vi "Periodic Tasks.vi"(8 "error in":errorcluster) -> ()   [LabVIEW 2014]
doc: "This VI runs in parallel to other tasks. It can contain as many user-defined periodic loops as you need. These can carry out PID or other sorts of timed response."
uses:
  <vilib>/Rock Robotics/SystemInterfaces/Utilities/FPGA_UtilitiesLED Source.ctl
  <vilib>/Rock Robotics/SystemInterfaces/Utilities/FPGA_UtilitiesLED State.ctl
  Robot Global Data.vi
  <vilib>/Rock Robotics/WPI/Relay/WPI_RelayValue.ctl
panel:
  out "Encoder Alarm Statuses":string[](array[string])
  out "Directions":string[](array[string])
  out "Velocities":dbl[](array[numeric])
  out "Encoder Distances":dbl[](array[numeric])
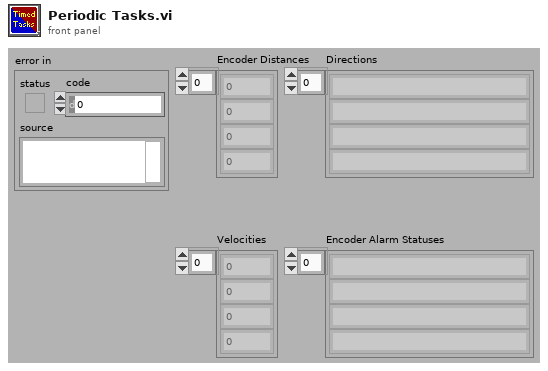
[diagram p1: front panel]
types:
  T1 = enum16{"open", "replace", "create", "open or create", "replace or create", "replace or create with confirmation"}
  T2 = typedef "WPI_DigitalInputDevRef.ctl" = cluster{"DevStatus":errorcluster, "DIO Channel":T3, "Digital Module":T4}
  T3 = typedef "FPGA_DIOChannel.ctl" = enum8{"DIO 1", "DIO 2", "DIO 3", "DIO 4", "DIO 5", "DIO 6", "DIO 7", "DIO 8", "DIO 9", "DIO 10", "DIO 11", "DIO 12", "DIO 13", "DIO 14", "Invalid"}
  T4 = typedef "FPGA_TypedefDigitalModule.ctl" = enum16{"Digital Module 1", "Digital Module 2"}
  T5 = typedef "WPI_RelayValue.ctl" = enum16{"Off", "On", "Forward", "Reverse"}
  T6 = typedef "WPI_RelayDevRef.ctl" = cluster{"DevStatus":errorcluster, "Relay Channel":T7, "Digital Module":T4, "Relay Direction":T8}
  T7 = typedef "FPGA_DIORelayChannel.ctl" = enum8{"Relay 1", "Relay 2", "Relay 3", "Relay 4", "Relay 5", "Relay 6", "Relay 7", "Relay 8", "Invalid"}
  T8 = typedef "WPI_RelayDirection.ctl" = enum16{"Both directions", "Forward only", "Reverse only"}
  T9 = typedef "FPGA_UtilitiesLED State.ctl" = enum16{"Off", "On", "Toggle"}
  T10 = typedef "FPGA_UtilitiesLED Source.ctl" = enum16{"User LED", "FPGA LED"}
  T11 = typedef "WPI_AnalogChannelDevRef.ctl" = cluster{"DevStatus":errorcluster, "Analog Module":T12, "Analog Channel":T13}
  T12 = typedef "FPGA_TypedefAnalogModule.ctl" = enum16{"Analog Module 1", "Analog Module 2"}
  T13 = typedef "FPGA_AIChannel.ctl" = enum8{"AI 1", "AI 2", "AI 3", "AI 4", "AI 5", "AI 6", "AI 7", "AI 8", "Invalid"}
  T14 = typedef "WPI_GyroDevRef.ctl" = cluster{"DevStatus":errorcluster, "Analog Module":T12, "Analog Channel":T13, "Offset":dbl, "Gain (VoltsPerDegree/Second)":dbl}
  T15 = typedef "WPI_CompressorDevRef.ctl" = cluster{"DevStatus":errorcluster, "DigitalInputDevRef":T2, "RelayDevRef":T6}
  T16 = typedef "WPI_EncoderDevRef.ctl" = cluster{"DevStatus":errorcluster, "EncoderIndex":T17, "CounterIndex":T18, "DistancePerCount":dbl, "Decoding Type":T19}
  T17 = typedef "FPGA_EncoderIdx.ctl" = enum8{"Enc 0", "Enc 1", "Enc 2", "Enc 3", "Invalid"}
  T18 = typedef "FPGA_CounterCtrSystemIndex.ctl" = enum8{"Ctr 0", "Ctr 1", "Ctr 2", "Ctr 3", "Ctr 4", "Ctr 5", "Ctr 6", "Ctr 7", "Invalid"}
  T19 = typedef "WPI_EncoderType.ctl" = enum16{"1x", "2x", "4x"}
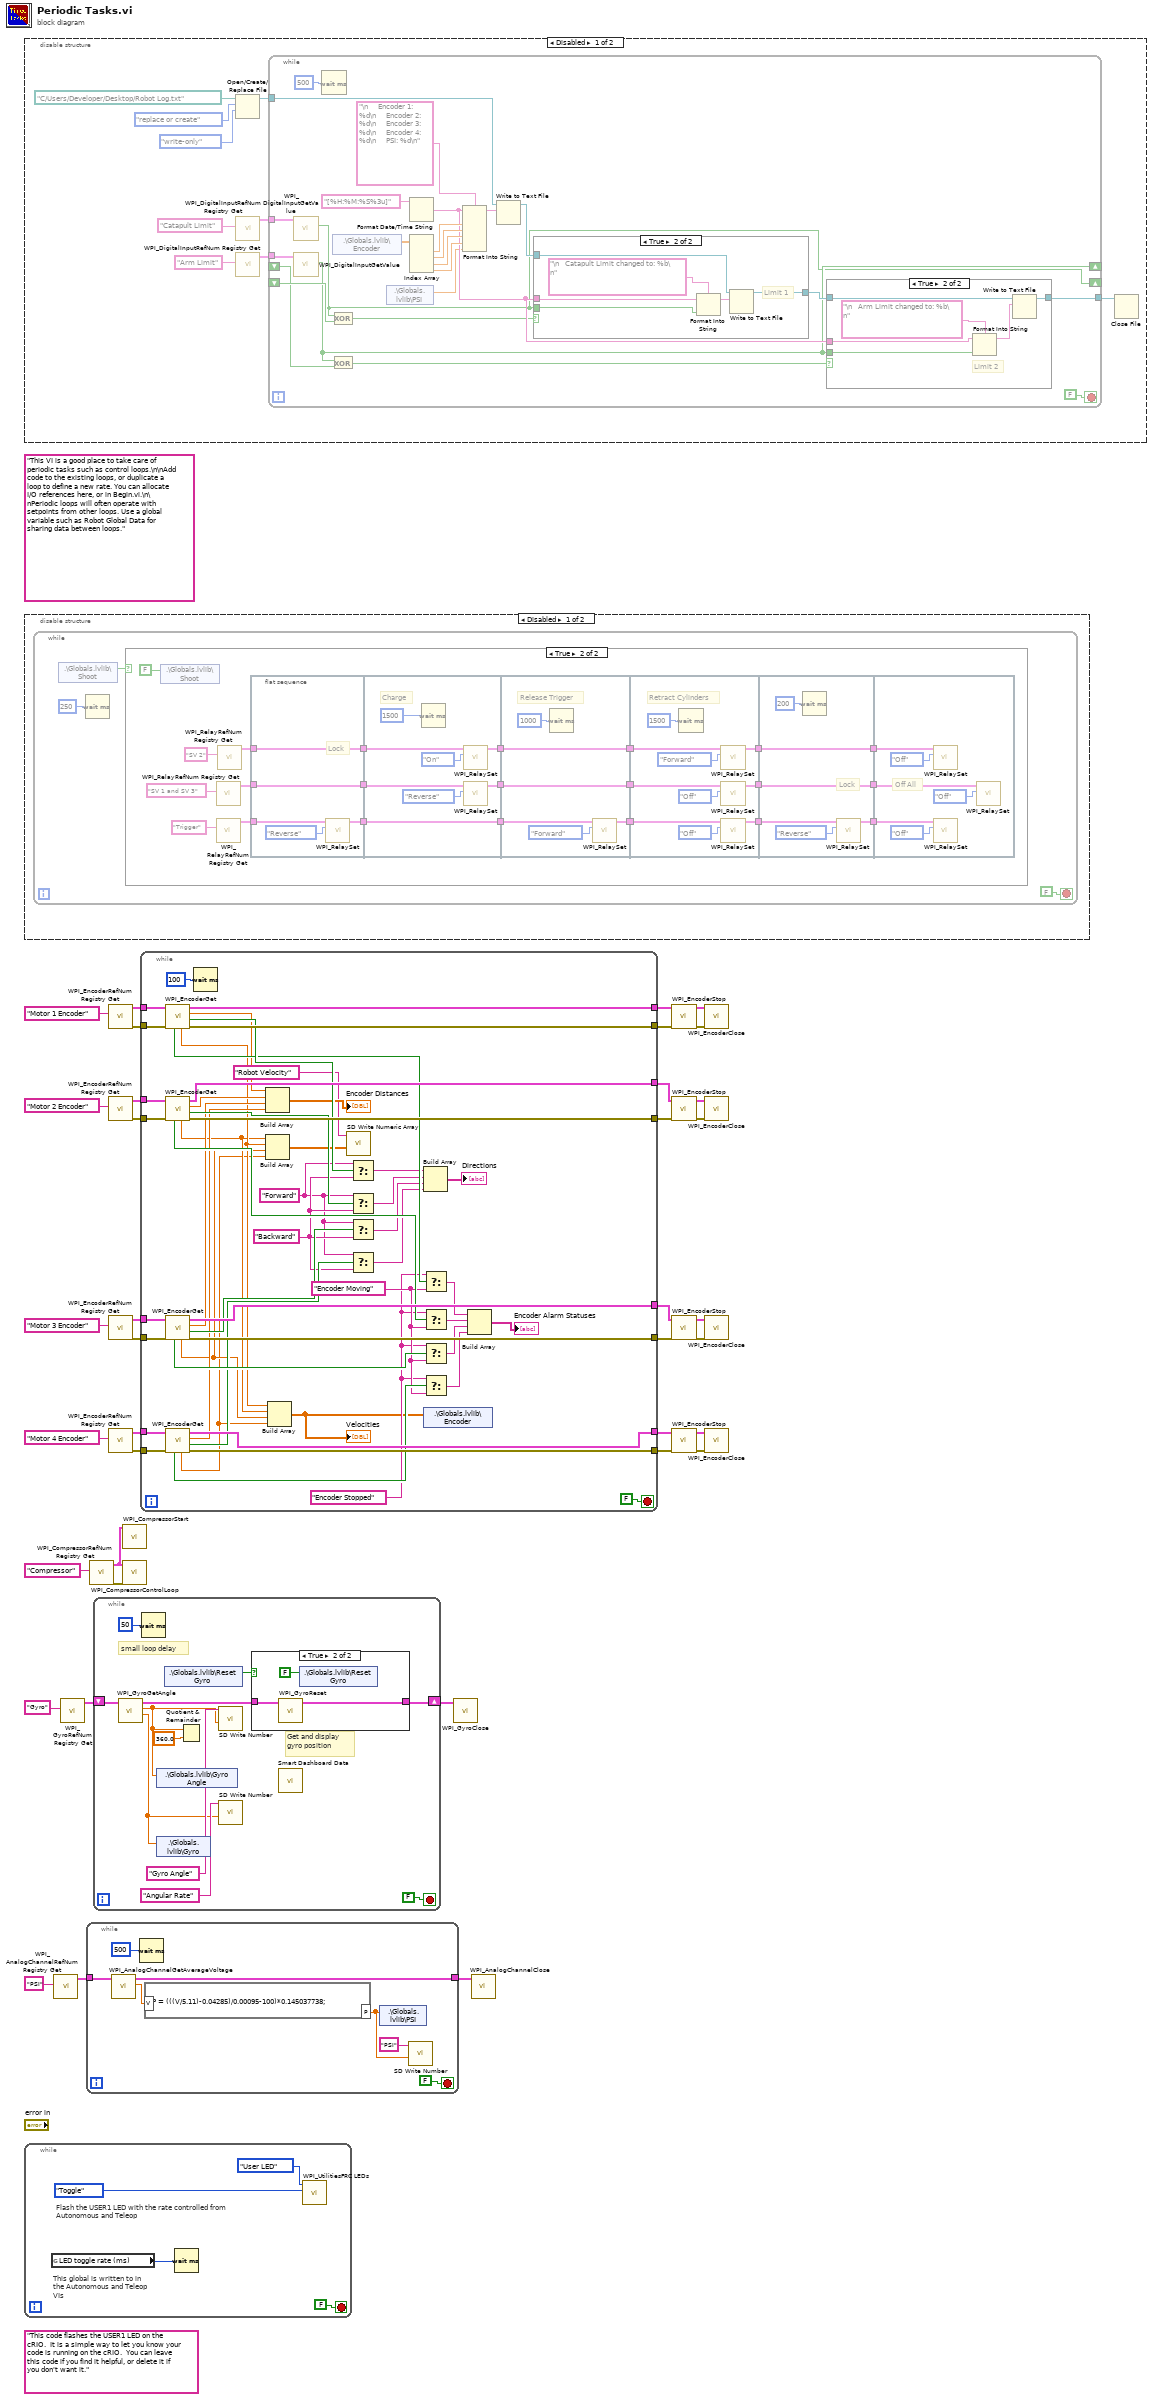
[diagram p0: block diagram]
diagram:
  (unwired) "This code flashes the USER1 LED on the cRIO.  It is a simple way to let you know your code is running on the cRIO.  You can leave this code if you find it helpful, or delete it if you don't want it."
  (unwired) "This VI is a good place to take care of periodic tasks such as control loops.\n\nAdd code to the existing loops, or duplicate a loop to define a new rate. You can allocate I/O references here, or in Begin.vi.\n\nPeriodic loops will often operate with setpoints from other loops. Use a global variable such as Robot Global Data for sharing data between loops."
  n1 = disable-structure shown="Disabled" {
    frame Disabled {
      n2 = Open/Create/Replace File(file path (use dialog)=path "C:/Users/Developer/Desktop/Robot Log.txt", operation (0:open)=T1."replace or create", access (0:read/write)=enum16{"read/write", "read-only", "write-only"}."write-only") -> (refnum out=w43:refnum<file>)  [unwired: 3 in, 2 out]
      n3 = call <vilib>:"WPI_DigitalInputRefNum Registry Get.vi"("refnum name"="Catapult Limit") -> ("DigitalInputDevRef"=w38:T2)  [unwired: 9 in, 1 out]
      n4 = call <vilib>:"WPI_DigitalInputRefNum Registry Get.vi"("refnum name"="Arm Limit") -> ("DigitalInputDevRef"=w39:T2)  [unwired: 9 in, 1 out]
      n5 = while {
        tunnel: w43 -> [w66]
        tunnel: [w55] -> w42
        shift-right: [w51] -> _
        shift-left: _ -> [w58]
        shift-right: [w50] -> _
        shift-left: _ -> [w59]
        tunnel: w39 -> [w49]
        tunnel: w38 -> [w48]
        stop <- FALSE stop-if-true
        n6 = call <vilib>:"WPI_DigitalInputGetValue.vi"("DigitalInputDevRef"=w48) -> ("Value"=w50:bool)  [unwired: 8 in, 2 out]
        n7 = call <vilib>:"WPI_DigitalInputGetValue.vi"("DigitalInputDevRef"=w49) -> ("Value"=w51:bool)  [unwired: 8 in, 2 out]
        n8 = Wait (ms)(milliseconds to wait=u32 500) -> ()  [unwired: 1 out]
        n9 = Exclusive Or(1:w59, 2:w50) -> (0:w53:bool)
        n10 = Exclusive Or(1:w58, 2:w51) -> (0:w52:bool)
        n11 = shared-variable ".\\Globals.lvlib\\Encoder"() -> (w64:dbl[])  [unwired: 1 in, 1 out]
        n12 = shared-variable ".\\Globals.lvlib\\PSI"() -> (w47:dbl)  [unwired: 1 in, 1 out]
        n13 = Format Date/Time String(time format string (%c)="[%H:%M:%S%3u]") -> (date/time string=w54:string)  [unwired: 2 in]
        n14 = Index Array(array=w64) -> (element #1=w63:dbl, element #2=w62:dbl, element #3=w61:dbl, element #4=w60:dbl)  [unwired: 4 in]
        n15 = Format Into String(format string="\n     Encoder 1: %d\n     Encoder 2: %d\n     Encoder 3: %d\n     Encoder 4: %d\n     PSI: %d\n", initial string=w54, w63, w62, w61, w60, w47) -> (resulting string=w67:string)  [unwired: 1 in, 1 out]
        n16 = Write to Text File(file (use dialog)=w66, text=w67) -> (refnum out=w57:refnum<file>)  [unwired: 2 in, 2 out]
        n17 = case shown="True" w53 {
          tunnel: w50 -> [_ w84]
          tunnel: w57 -> [w78 w83]
          tunnel: [w78 w82] -> w56
          tunnel: w54 -> [_ w81]
          frame False {
          }
          frame True {
            # "Limit 1"
            n18 = Format Into String(format string="\n   Catapult Limit changed to: %b\n", initial string=w81, w84) -> (resulting string=w79:string)  [unwired: 1 in, 1 out]
            n19 = Write to Text File(file (use dialog)=w83, text=w79) -> (refnum out=w82:refnum<file>)  [unwired: 2 in, 2 out]
          }
        }
        n20 = case shown="True" w52 {
          tunnel: w51 -> [_ w77]
          tunnel: w56 -> [w71 w76]
          tunnel: [w71 w75] -> w55
          tunnel: w54 -> [_ w74]
          frame False {
          }
          frame True {
            # "Limit 2"
            n21 = Format Into String(format string="\n   Arm Limit changed to: %b\n", initial string=w74, w77) -> (resulting string=w72:string)  [unwired: 1 in, 1 out]
            n22 = Write to Text File(file (use dialog)=w76, text=w72) -> (refnum out=w75:refnum<file>)  [unwired: 2 in, 2 out]
          }
        }
      }
      n23 = Close File(refnum=w42) -> ()  [unwired: 1 in, 2 out]
    }
    frame Enabled {
    }
  }
  n24 = disable-structure shown="Disabled" {
    frame Disabled {
      n25 = while {
        stop <- FALSE stop-if-true
        n26 = shared-variable ".\\Globals.lvlib\\Shoot"() -> (w86:bool)  [unwired: 1 in, 1 out]
        n27 = Wait (ms)(milliseconds to wait=u32 250) -> ()  [unwired: 1 out]
        n28 = case shown="True" w86 {
          frame False {
          }
          frame True {
            n29 = shared-variable ".\\Globals.lvlib\\Shoot"(FALSE ("Shoot")) -> ()  [unwired: 1 in, 1 out]
            n30 = call <vilib>:"WPI_RelayRefNum Registry Get.vi"("refnum name"="SV 1 and SV 3") -> ("RelayDevRef"=w104:T6)  [unwired: 9 in, 1 out]
            n31 = call <vilib>:"WPI_RelayRefNum Registry Get.vi"("refnum name"="Trigger") -> ("RelayDevRef"=w105:T6)  [unwired: 9 in, 1 out]
            n32 = call <vilib>:"WPI_RelayRefNum Registry Get.vi"("refnum name"="SV 2") -> ("RelayDevRef"=w106:T6)  [unwired: 9 in, 1 out]
            n33 = flat-sequence {
              tunnel: w106 -> [w112]
              tunnel: w105 -> [w113]
              tunnel: w104 -> [w111]
              tunnel: [w112] -> w103
              tunnel: [w111] -> w102
              tunnel: [w110] -> w101
              tunnel: w103 -> [w121]
              tunnel: w102 -> [w119]
              tunnel: w101 -> [w118]
              tunnel: [w118] -> w100
              tunnel: [w116] -> w98
              tunnel: [w115] -> w96
              tunnel: w100 -> [w127]
              tunnel: [w125] -> w99
              tunnel: w98 -> [w124]
              tunnel: [w124] -> w97
              tunnel: w96 -> [w123]
              tunnel: [w123] -> w95
              tunnel: w99 -> [w136]
              tunnel: w97 -> [w134]
              tunnel: w95 -> [w132]
              tunnel: [w131] -> w94
              tunnel: [w130] -> w93
              tunnel: [w129] -> w90
              tunnel: w94 -> [w144]
              tunnel: w93 -> [w142]
              tunnel: [w142] -> w92
              tunnel: [w141] -> w91
              tunnel: w90 -> [w141]
              tunnel: [w140] -> w89
              tunnel: w92 -> [w147]
              tunnel: w91 -> [w146]
              tunnel: w89 -> [w145]
              frame #0 {
                # "Lock"
                n34 = call <vilib>:"WPI_RelaySet.vi"("RelayValue"=WPI_RelayValue."Reverse", "RelayDevRef"=w113) -> ("RelayDevRef"=w110:T6)  [unwired: 8 in, 1 out]
              }
              frame #1 {
                # "Charge"
                n35 = Wait (ms)(milliseconds to wait=u32 1500) -> ()  [unwired: 1 out]
                n36 = call <vilib>:"WPI_RelaySet.vi"("RelayValue"=WPI_RelayValue."On", "RelayDevRef"=w121) -> ("RelayDevRef"=w115:T6)  [unwired: 8 in, 1 out]
                n37 = call <vilib>:"WPI_RelaySet.vi"("RelayValue"=WPI_RelayValue."Reverse", "RelayDevRef"=w119) -> ("RelayDevRef"=w116:T6)  [unwired: 8 in, 1 out]
              }
              frame #2 {
                # "Release Trigger"
                n38 = Wait (ms)(milliseconds to wait=u32 1000) -> ()  [unwired: 1 out]
                n39 = call <vilib>:"WPI_RelaySet.vi"("RelayValue"=WPI_RelayValue."Forward", "RelayDevRef"=w127) -> ("RelayDevRef"=w125:T6)  [unwired: 8 in, 1 out]
              }
              frame #3 {
                # "Retract Cylinders"
                n40 = Wait (ms)(milliseconds to wait=u32 1500) -> ()  [unwired: 1 out]
                n41 = call <vilib>:"WPI_RelaySet.vi"("RelayValue"=WPI_RelayValue."Forward", "RelayDevRef"=w132) -> ("RelayDevRef"=w129:T6)  [unwired: 8 in, 1 out]
                n42 = call <vilib>:"WPI_RelaySet.vi"("RelayValue"=WPI_RelayValue."Off", "RelayDevRef"=w134) -> ("RelayDevRef"=w130:T6)  [unwired: 8 in, 1 out]
                n43 = call <vilib>:"WPI_RelaySet.vi"("RelayValue"=WPI_RelayValue."Off", "RelayDevRef"=w136) -> ("RelayDevRef"=w131:T6)  [unwired: 8 in, 1 out]
              }
              frame #4 {
                # "Lock"
                n44 = Wait (ms)(milliseconds to wait=u32 200) -> ()  [unwired: 1 out]
                n45 = call <vilib>:"WPI_RelaySet.vi"("RelayValue"=WPI_RelayValue."Reverse", "RelayDevRef"=w144) -> ("RelayDevRef"=w140:T6)  [unwired: 8 in, 1 out]
              }
              frame #5 {
                # "Off All"
                n46 = call <vilib>:"WPI_RelaySet.vi"("RelayValue"=WPI_RelayValue."Off", "RelayDevRef"=w146) -> ()  [unwired: 8 in, 2 out]
                n47 = call <vilib>:"WPI_RelaySet.vi"("RelayValue"=WPI_RelayValue."Off", "RelayDevRef"=w145) -> ()  [unwired: 8 in, 2 out]
                n48 = call <vilib>:"WPI_RelaySet.vi"("RelayValue"=WPI_RelayValue."Off", "RelayDevRef"=w147) -> ()  [unwired: 8 in, 2 out]
              }
            }
          }
        }
      }
    }
    frame Enabled {
    }
  }
  n49 = while {
    stop <- FALSE stop-if-true
    # "This global is written to in the Autonomous and Teleop VIs"
    # "Flash the USER1 LED with the rate controlled from Autonomous and Teleop"
    n50 = global read "Robot Global Data.vi" "LED toggle rate (ms)"() -> (w151:u32)
    n51 = Wait (ms)(milliseconds to wait=w151) -> ()  [unwired: 1 out]
    n52 = call <vilib>:"WPI_UtilitiesFRC LEDs.vi"("State"=FPGA_UtilitiesLED_State."Toggle", "LED Type"=FPGA_UtilitiesLED_Source."User LED") -> ()  [unwired: 1 in, 9 out]
  }
  n53 = call <vilib>:"WPI_AnalogChannelRefNum Registry Get.vi"("refnum name"="PSI") -> ("AIDeviceRef"=w2:T11)  [unwired: 9 in, 1 out]
  n54 = call <vilib>:"WPI_GyroRefNum Registry Get.vi"("refnum name"="Gyro") -> ("GyroDevRef"=w37:T14)  [unwired: 9 in, 1 out]
  n55 = while {
    tunnel: w2 -> [w160]
    tunnel: [w156] -> w1
    stop <- FALSE stop-if-true
    n56 = call <vilib>:"WPI_AnalogChannelGetAverageVoltage.vi"("AIDeviceRef"=w160) -> ("Voltage"=w159:dbl, "AIDeviceRef"=w156:T11)  [unwired: 8 in, 1 out]
    n57 = Wait (ms)(milliseconds to wait=u32 500) -> ()  [unwired: 1 out]
    n58 = formula code="P = (((V/5.11)-0.04285)/0.00095-100)*0.145037738;"("V"=w159) -> ("P"=w157:dbl)
    n59 = shared-variable ".\\Globals.lvlib\\PSI"(w157) -> ()  [unwired: 1 in, 1 out]
    n60 = call <vilib>:"SD Write Number.vi"("Numeric"=w157, "Name"="PSI") -> ()  [unwired: 8 in, 2 out]
  }
  n61 = call <vilib>:"WPI_CompressorRefNum Registry Get.vi"("refnum name"="Compressor") -> ("error out"=w5:errorcluster, "CompressorDevRef"=w6:T15)  [unwired: 9 in]
  n62 = while {
    shift-right: [w167] -> w35
    shift-left: w37 -> [w169]
    stop <- FALSE stop-if-true
    # "small loop delay"
    # "Get and display\ngyro position"
    n63 = call <vilib>:"WPI_GyroGetAngle.vi"("GyroDevRef"=w169) -> ("Angular Rate"=w163:dbl, "Angle"=w162:dbl, "GyroDevRef"=w168:T14)  [unwired: 1 in, 7 out]
    n64 = Wait (ms)(milliseconds to wait=u32 50) -> ()  [unwired: 1 out]
    n65 = shared-variable ".\\Globals.lvlib\\Gyro Angle"(w162) -> ()  [unwired: 1 in, 1 out]
    n66 = shared-variable ".\\Globals.lvlib\\Gyro"(w163) -> ()  [unwired: 1 in, 1 out]
    n67 = shared-variable ".\\Globals.lvlib\\Reset Gyro"() -> (w166:bool)  [unwired: 1 in, 1 out]
    n68 = Quotient & Remainder(x=w162, y=360.0) -> ()  [unwired: 2 out]
    n69 = call <vilib>:"SD Write Number.vi"("Numeric"=w162, "Name"="Gyro Angle") -> ()  [unwired: 8 in, 2 out]
    n70 = call <vilib>:"SD Write Number.vi"("Numeric"=w163, "Name"="Angular Rate") -> ()  [unwired: 8 in, 2 out]
    n71 = case shown="True" w166 {
      tunnel: w168 -> [w173 w176]
      tunnel: [w173 w175] -> w167
      frame False {
      }
      frame True {
        n72 = call <vilib>:"WPI_GyroReset.vi"("GyroDevRef"=w176) -> ("GyroDevRef"=w175:T14)  [unwired: 9 in, 1 out]
        n73 = shared-variable ".\\Globals.lvlib\\Reset Gyro"(FALSE ("Reset Gyro")) -> ()  [unwired: 1 in, 1 out]
      }
    }
    n74 = call "Smart Dashboard Data.vi"() -> ()  [unwired: 12 in]
  }
  n75 = call <vilib>:"WPI_EncoderRefNum Registry Get.vi"("refnum name"="Motor 1 Encoder") -> ("error out"=w33:errorcluster, "EncoderDevRef"=w34:T16)  [unwired: 9 in]
  n76 = call <vilib>:"WPI_EncoderRefNum Registry Get.vi"("refnum name"="Motor 2 Encoder") -> ("error out"=w30:errorcluster, "EncoderDevRef"=w29:T16)  [unwired: 9 in]
  n77 = call <vilib>:"WPI_EncoderRefNum Registry Get.vi"("refnum name"="Motor 3 Encoder") -> ("error out"=w27:errorcluster, "EncoderDevRef"=w28:T16)  [unwired: 9 in]
  n78 = call <vilib>:"WPI_EncoderRefNum Registry Get.vi"("refnum name"="Motor 4 Encoder") -> ("error out"=w8:errorcluster, "EncoderDevRef"=w7:T16)  [unwired: 9 in]
  n79 = call <vilib>:"WPI_CompressorStart.vi"("CompressorDevRef"=w6) -> ()  [unwired: 9 in, 2 out]
  n80 = call <vilib>:"WPI_CompressorControlLoop.vi"("error in (no error)"=w5, "CompressorDevRef"=w6) -> ()  [unwired: 10 in]
  n81 = while {
    tunnel: w34 -> [w228]
    tunnel: w33 -> [w227]
    tunnel: w30 -> [w226]
    tunnel: w29 -> [w225]
    tunnel: w28 -> [w224]
    tunnel: w27 -> [w223]
    tunnel: [w222] -> w25
    tunnel: [w221] -> w22
    tunnel: [w220] -> w18
    tunnel: [w219] -> w17
    tunnel: [w218] -> w16
    tunnel: [w217] -> w14
    tunnel: [w216] -> w13
    tunnel: [w215] -> w10
    tunnel: w8 -> [w214]
    tunnel: w7 -> [w213]
    stop <- FALSE stop-if-true
    w201 = "Backward" ("f")
    w202 = "Encoder Moving" ("f")
    w199 = "Encoder Stopped"
    w200 = "Forward"
    n82 = call <vilib>:"WPI_EncoderGet.vi"("error in (no error)"=w227, "EncoderDevRef"=w228) -> ("error out"=w220:errorcluster, "Direction"=w207:bool, "Distance"=w198:dbl, "EncoderDevRef"=w222:T16, "Rate"=w193:dbl, "Stopped"=w206:bool)  [unwired: 4 out]
    n83 = call <vilib>:"WPI_EncoderGet.vi"("error in (no error)"=w226, "EncoderDevRef"=w225) -> ("error out"=w218:errorcluster, "Direction"=w205:bool, "Distance"=w197:dbl, "EncoderDevRef"=w219:T16, "Rate"=w192:dbl, "Stopped"=w204:bool)  [unwired: 4 out]
    n84 = call <vilib>:"WPI_EncoderGet.vi"("error in (no error)"=w223, "EncoderDevRef"=w224) -> ("error out"=w217:errorcluster, "Direction"=w211:bool, "Distance"=w196:dbl, "EncoderDevRef"=w221:T16, "Rate"=w191:dbl, "Stopped"=w210:bool)  [unwired: 4 out]
    n85 = call <vilib>:"WPI_EncoderGet.vi"("error in (no error)"=w214, "EncoderDevRef"=w213) -> ("error out"=w216:errorcluster, "Direction"=w209:bool, "Distance"=w195:dbl, "EncoderDevRef"=w215:T16, "Rate"=w177:dbl, "Stopped"=w208:bool)  [unwired: 4 out]
    n86 = Wait (ms)(milliseconds to wait=u32 100) -> ()  [unwired: 1 out]
    n87 = Build Array(w198, w197, w196, w195) -> (→"Encoder Distances":dbl[])
    n88 = Build Array(w192, w193, w191, w177) -> (w180:dbl[])
    n89 = Build Array(w193, w192, w191, w177) -> (w178:dbl[])
    "Velocities" <- w178
    n90 = call <vilib>:"SD Write Numeric Array.vi"("Numeric Array"=w180, "Name"="Robot Velocity") -> ()  [unwired: 8 in, 2 out]
    n91 = Select(t=w200, s=w207, f=w201) -> (s? t:f=w190:string)
    n92 = Select(t=w200, s=w205, f=w201) -> (s? t:f=w189:string)
    n93 = Select(t=w200, s=w211, f=w201) -> (s? t:f=w188:string)
    n94 = Select(t=w200, s=w209, f=w201) -> (s? t:f=w187:string)
    n95 = Build Array(w190, w189, w188, w187) -> (→"Directions":string[])
    n96 = Select(t=w199, s=w206, f=w202) -> (s? t:f=w184:string)
    n97 = Select(t=w199, s=w204, f=w202) -> (s? t:f=w183:string)
    n98 = Select(t=w199, s=w210, f=w202) -> (s? t:f=w182:string)
    n99 = Select(t=w199, s=w208, f=w202) -> (s? t:f=w181:string)
    n100 = shared-variable ".\\Globals.lvlib\\Encoder"(w178) -> ()  [unwired: 1 in, 1 out]
    n101 = Build Array(w184, w183, w182, w181) -> (→"Encoder Alarm Statuses":string[])
  }
  n102 = call <vilib>:"WPI_GyroClose.vi"("GyroDevRef"=w35) -> ()  [unwired: 1 in, 10 out]
  n103 = call <vilib>:"WPI_AnalogChannelClose.vi"("AIDeviceRef"=w1) -> ()  [unwired: 10 in, 1 out]
  n104 = call <vilib>:"WPI_EncoderStop.vi"("error in (no error)"=w18, "EncoderDevRef"=w25) -> ("error out"=w19:errorcluster, "EncoderDevRef"=w24:T16)  [unwired: 8 in]
  n105 = call <vilib>:"WPI_EncoderStop.vi"("error in (no error)"=w16, "EncoderDevRef"=w17) -> ("error out"=w15:errorcluster, "EncoderDevRef"=w23:T16)  [unwired: 8 in]
  n106 = call <vilib>:"WPI_EncoderStop.vi"("error in (no error)"=w14, "EncoderDevRef"=w22) -> ("error out"=w21:errorcluster, "EncoderDevRef"=w20:T16)  [unwired: 8 in]
  n107 = call <vilib>:"WPI_EncoderStop.vi"("error in (no error)"=w13, "EncoderDevRef"=w10) -> ("error out"=w11:errorcluster, "EncoderDevRef"=w12:T16)  [unwired: 8 in]
  n108 = call <vilib>:"WPI_EncoderClose.vi"("error in (no error)"=w19, "EncoderDevRef"=w24) -> ()  [unwired: 9 in, 1 out]
  n109 = call <vilib>:"WPI_EncoderClose.vi"("error in (no error)"=w15, "EncoderDevRef"=w23) -> ()  [unwired: 9 in, 1 out]
  n110 = call <vilib>:"WPI_EncoderClose.vi"("error in (no error)"=w21, "EncoderDevRef"=w20) -> ()  [unwired: 9 in, 1 out]
  n111 = call <vilib>:"WPI_EncoderClose.vi"("error in (no error)"=w11, "EncoderDevRef"=w12) -> ()  [unwired: 9 in, 1 out]
